vi "Channel Registry.vi"(7 "New Channel Class":refnum<class "Pub Sub Message Channel.lvclass">, 10 "Action":T2(ring), 11 "Topic":string) -> (1 "Registered Channels":T1(c390), 2 "topic not found?":bool, 3 "Pub Sub Message Channel":refnum<class "Pub Sub Message Channel.lvclass">)   [LabVIEW 2020, in "Actor Pub Sub Channels.lvlib"]
uses:
  Actor Pub Sub Channels.lvlib
  Pub Sub Message Channel/Pub Sub Message Channel.lvclass
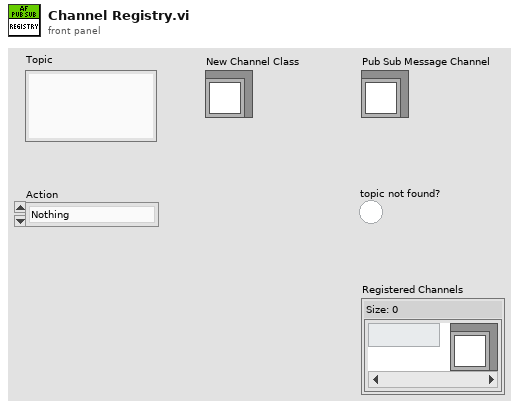
[diagram p1: front panel]
types:
  T1 = map{string, refnum<class "Pub Sub Message Channel.lvclass">}
  T2 = enum16{"Nothing", "Get Channel", "Get Or Create Channel", "Close Channel", "Dispose"}
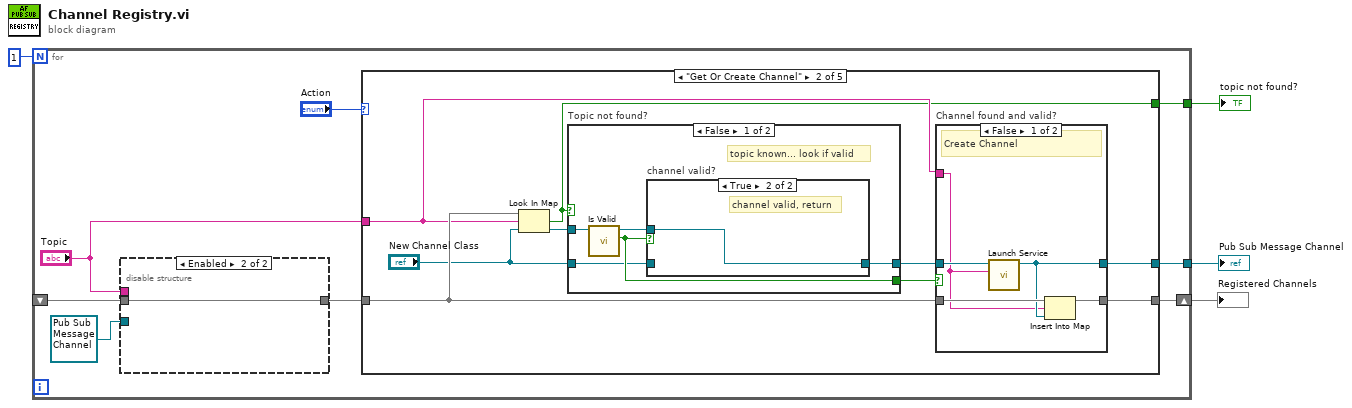
[diagram p0: block diagram]
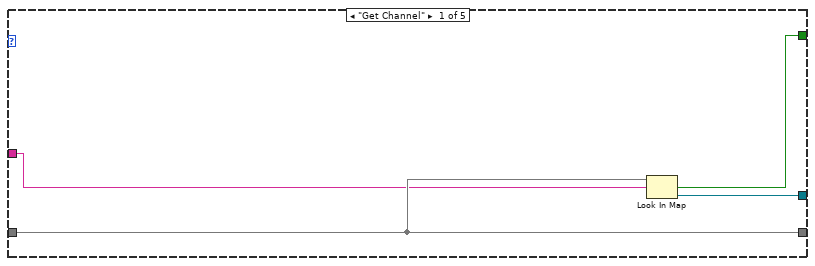
[diagram p2: hidden frame]
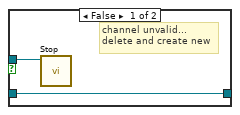
[diagram p3: hidden frame]
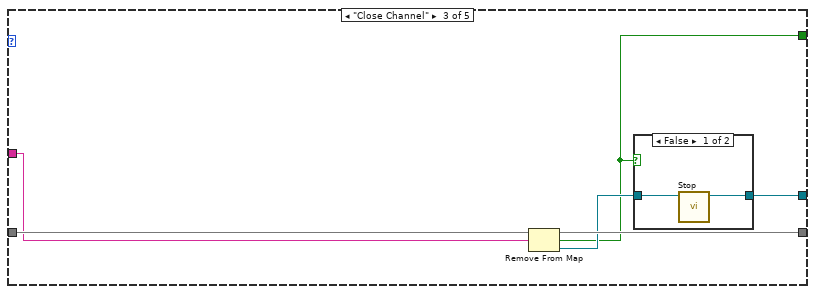
[diagram p6: hidden frame]
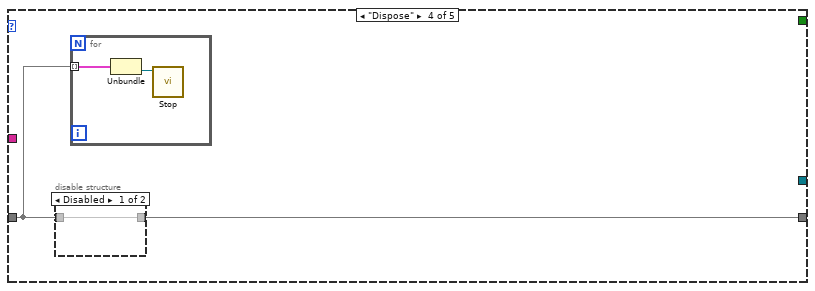
[diagram p8: hidden frame]
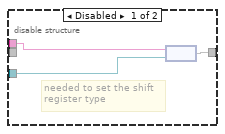
[diagram p11: hidden frame]
diagram:
  n1 = for {
    N: 1 -> [_]
    shift-right: [w10] -> w2
    shift-left: _ -> [w11]
    tunnel: [w9] -> w3
    tunnel: [w7] -> w1
    n2 = disable-structure shown="Enabled" {
      disable-tunnel: "Topic" -> [w59 _]
      disable-tunnel: [w58 w60] -> w12
      disable-tunnel: w11 -> [_ w60]
      disable-tunnel: refnum<class "Pub Sub Message Channel.lvclass"> refnum ("Pub Sub Message Channel out") -> [w57 _]
      frame Disabled {
        # "needed to set the shift \nregister type"
        n3 = node(w59, w57) -> (w58:T1)
      }
      frame Enabled {
      }
    }
    n4 = case shown="\"Get Or Create Channel\"" "Action" {
      tunnel: "Topic" -> [w14 w22 w45 _ _]
      tunnel: w12 -> [w15 w23 w47 w51 w56]
      tunnel: [w15 w25 w46 w52 w56] -> w10
      tunnel: [w16 w24 w43 _ _] -> w9
      tunnel: [w13 w19 w42 _ _] -> w7
      frame "Get Channel" {
        n5 = Look In Map(map=w15, key=w14) -> (key not found?=w13:bool, value=w16:refnum<class "Pub Sub Message Channel.lvclass">)  [unwired: 1 in]
      }
      frame "Get Or Create Channel" {
        n6 = Look In Map(map=w23, key=w22, default value="New Channel Class") -> (key not found?=w19:bool, value=w21:refnum<class "Pub Sub Message Channel.lvclass">)
        n7 = case "Topic not found?" shown="False" w19 {
          tunnel: w21 -> [w30 w34]
          tunnel: [w27 w34] -> w20
          tunnel: [w29 _] -> w18
          tunnel: "New Channel Class" -> [w26 _]
          frame False {
            # "topic known... look if valid"
            n8 = call "Is Valid.vi"("Pub Sub Message Channel in"=w30) -> ("Valid"=w29:bool, "Pub Sub Message Channel out"=w28:refnum<class "Pub Sub Message Channel.lvclass">)  [unwired: 8 in, 1 out]
            n9 = case "channel valid?" shown="True" w29 {
              tunnel: w28 -> [w32 w33]
              tunnel: [w31 w33] -> w27
              tunnel: w26 -> [w31 _]
              frame False {
                # "channel unvalid...\ndelete and create new"
                n10 = call "Stop.vi"("Pub Sub Message Channel in"=w32) -> ()  [unwired: 9 in, 2 out]
              }
              frame True {
                # "channel valid, return"
              }
            }
          }
          frame True {
            # "Topic unknown... \njust create"
          }
        }
        n11 = case "Channel found and valid?" shown="False" w18 {
          tunnel: [w39 w40] -> w25
          tunnel: [w36 w41] -> w24
          tunnel: w23 -> [w37 w40]
          tunnel: w22 -> [w35 _]
          tunnel: w20 -> [w38 w41]
          frame False {
            # "Create Channel"
            n12 = call "Launch Service.vi"("Topic"=w35, "Pub Sub Message Channel"=w38) -> ("Pub Sub Message Channel Out"=w36:refnum<class "Pub Sub Message Channel.lvclass">)  [unwired: 8 in, 1 out]
            n13 = Insert Into Map(map in=w37, key=w35, value=w36) -> (map out=w39:T1)  [unwired: 2 out]
          }
          frame True {
            # "Get existing"
          }
        }
      }
      frame "Close Channel" {
        n14 = Remove From Map(10:w45, 11:w47) -> (1:w44:refnum<class "Pub Sub Message Channel.lvclass">, 2:w42:bool, 3:w46:T1)
        n15 = case shown="False" w42 {
          tunnel: w44 -> [w49 w50]
          tunnel: [w48 w50] -> w43
          frame False {
            n16 = call "Stop.vi"("Pub Sub Message Channel in"=w49) -> ("Pub Sub Message Channel out"=w48:refnum<class "Pub Sub Message Channel.lvclass">)  [unwired: 9 in, 1 out]
          }
          frame True {
          }
        }
      }
      frame "Dispose" {
        n17 = disable-structure shown="Disabled" {
          disable-tunnel: [w55 _] -> w52
          disable-tunnel: w51 -> [w55 _]
          frame Disabled {
          }
          frame Enabled {
          }
        }
        n18 = for {
          tunnel: w51 -> [w54] mode=indexing
          n19 = Unbundle(w54) -> ("Pub Sub Message Channel out"=w53:refnum<class "Pub Sub Message Channel.lvclass">)  [unwired: 1 out]
          n20 = call "Stop.vi"("Pub Sub Message Channel in"=w53) -> ()  [unwired: 9 in, 2 out]
        }
      }
      frame "Nothing" {
      }
    }
  }
  "Pub Sub Message Channel" <- w3
  "Registered Channels" <- w2
  "topic not found?" <- w1
